vi "Get Limit Plots.vi"(0 "Limits File Path":path, 5 "Limit Range (dB SPL)":dbl=5.0, 11 "error in (no error)":errorcluster) -> (4 "Positive Limit Plot":T1, 6 "Negative Limit Plot":T1, 15 "error out":errorcluster)   [LabVIEW 2020]
doc: "VI gest the positive and negative limit signals within the limit range from the standard signal obtained from reading the Limit file."
uses:
  Plot Data.ctl
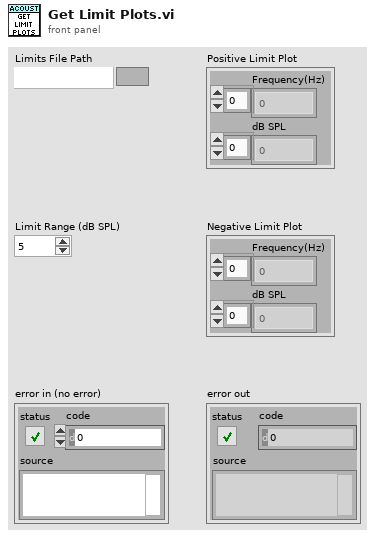
[diagram p1: front panel]
types:
  T1 = typedef "Plot Data.ctl" = cluster{"Frequency(Hz)":dbl[], "dB SPL":dbl[]}
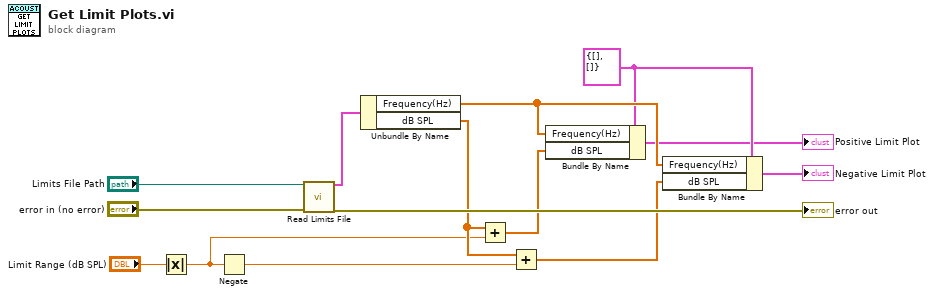
[diagram p0: block diagram]
diagram:
  w5 = T1 {"Frequency(Hz)"=[], "dB SPL"=[]} ("Ideal Data")
  n1 = Absolute Value(x="Limit Range (dB SPL)") -> (abs(x)=w1:dbl)
  n2 = Negate(x=w1) -> (-x=w9:dbl)
  n3 = call "Read Limits File.vi"("Limits File Path"="Limits File Path", "error in (no error)"="error in (no error)") -> ("Limit Data"=w11:T1, "error out"=→"error out":errorcluster)  [unwired: 12 in]
  n4 = Unbundle By Name(w11) -> ("Frequency(Hz)"=w7:dbl[], "dB SPL"=w10:dbl[])
  n5 = Add(x=w10, y=w1) -> (x+y=w8:dbl[])
  n6 = Add(x=w10, y=w9) -> (x+y=w6:dbl[])
  n7 = Bundle By Name(cluster=w5, "Frequency(Hz)"=w7, "dB SPL"=w8) -> (→"Positive Limit Plot":T1)
  n8 = Bundle By Name(cluster=w5, "Frequency(Hz)"=w7, "dB SPL"=w6) -> (→"Negative Limit Plot":T1)
